vi "Utility Default Instrument Setup.vi"(8 "error in (no error)":errorcluster, 11 "VISA resource name":refnum<visa-resource-name>) -> (0 "error out":errorcluster, 3 "VISA resource name out":refnum<visa-resource-name>)   [LabVIEW 2012, in "Quantum Composers 9000 Series.lvlib"]
doc: "This Utility VI sends a default command string to the instrument whenever a new VISA session is opened, or the instrument is reset. This VI is intended to be used as a subVI for the Initialize and Reset VI's. Altering this VI could cause these two VI's to operate incorrectly."
uses:
  Quantum Composers 9000 Series.lvlib
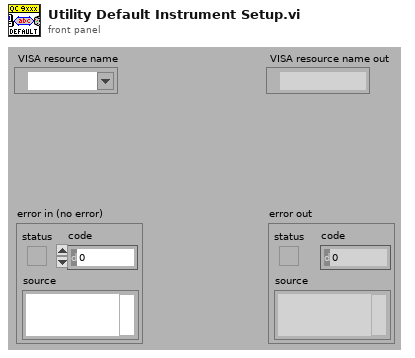
[diagram p1: front panel]
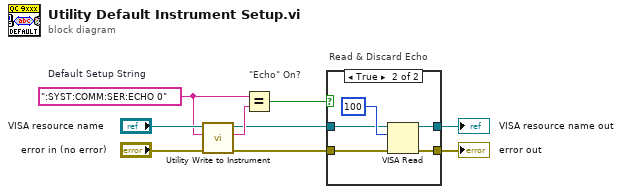
[diagram p0: block diagram]
diagram:
  w5 = ":SYST:COMM:SER:ECHO 0"  # Default Setup String
  # "\"Echo\" On?"
  # "Read & Discard Echo"
  n1 = call "Utility Write to Instrument.vi"("error in (no error)"="error in (no error)", "Write Buffer"=w5, "VISA resource name"="VISA resource name") -> ("error out"=w3:errorcluster, "Read Buffer"=w6:string, "VISA resource name out"=w4:refnum<visa-resource-name>)  [unwired: 6 in]
  n2 = Equal?(x=w5, y=w6) -> (x = y?=w7:bool)
  n3 = case shown="True" w7 {
    tunnel: w4 -> [w11 w12]
    tunnel: w3 -> [w10 w14]
    tunnel: [w11 w16] -> w1
    tunnel: [w10 w13] -> w2
    frame False {
    }
    frame True {
      n4 = VISA Read(VISA resource name=w12, byte count=u32 100 ("byte count (0)"), error in (no error)=w14) -> (VISA resource name out=w16:refnum<visa-resource-name>, error out=w13:errorcluster)  [unwired: 2 out]
    }
  }
  "error out" <- w2
  "VISA resource name out" <- w1
